vi "LED-Set Text_Tag.vi"() -> (0 "\"Set Text\" Label":string)   [LabVIEW 2010, in "LED Display.xctl"]
uses:
  LED Display.xctl
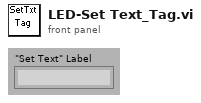
[diagram p1: front panel]
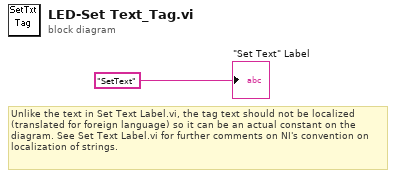
[diagram p0: block diagram]
diagram:
  # "Unlike the text in Set Text Label.vi, the tag text should not be localized (translated for foreign language) so it can be an actual constant on the diagram. See Set Text Label.vi for further comments on NI's convention on localization of strings."
  "\"Set Text\" Label" <- "SetText" ("String")
